vi "Loop_Overlord.vi"() -> ()   [LabVIEW 2017, in "Rotation_Overlord.lvlib"]
uses:
  Rotation_Overlord.lvlib
  CLUSTER_Rotation_CMD.ctl
  ENUM_Rotation_Positon.ctl
  TypeDef/CLUSTER_Overlord_Systems.ctl
  Arm/CLUSTER_CMD_SM_Lift_Rotate.ctl
  Arm/ENUM_SM_Rotate_Positions.ctl
  Claw Rotation/CLUSTER_CMD_SM_Lift_Rotate.ctl
  Claw Rotation/ENUM_SM_Rotate_Positions.ctl
  Lift/CLUSTER_CMD_SM_Lift_Rotate.ctl
  Lift/ENUM_SM_Rotate_Positions.ctl
  ENUM_Overloard_State.ctl
  Arm/ENUM_SM_State.ctl
  Claw Rotation/ENUM_SM_State.ctl
  Lift/ENUM_SM_State.ctl
  Lift/CLUSTER_ACT_Lift Output.ctl
  _SHARE ALL/RoboRio Share All/SRX Share All/TypeDefs SRX/Cluster_SRX_General Data.ctl
  _SHARE ALL/RoboRio Share All/SRX Share All/TypeDefs SRX/Cluster_SRX_Common Runtime Data.ctl
  _SHARE ALL/RoboRio Share All/SRX Share All/TypeDefs SRX/Cluster_SRX_Error Calculations.ctl
  _SHARE ALL/RoboRio Share All/SRX Share All/TypeDefs SRX/Cluster_SRX_Voltage Out Data.ctl
  _SHARE ALL/RoboRio Share All/SRX Share All/TypeDefs SRX/Cluster_SRX_Sensor Out Data.ctl
  _SHARE ALL/RoboRio Share All/SRX Share All/TypeDefs SRX/Cluster_SRX_Sensor Quad Data.ctl
  _SHARE ALL/RoboRio Share All/SRX Share All/TypeDefs SRX/Cluster_SRX_Analog In Data.ctl
  _SHARE ALL/RoboRio Share All/SRX Share All/TypeDefs SRX/Cluster_SRX_PWM Sensor Data.ctl
  _SHARE ALL/RoboRio Share All/SRX Share All/TypeDefs SRX/Cluster_SRX_F and R Limit Indicators.ctl
  ENUM_Overloard_Action.ctl
  _SHARE ALL/Global Share All/Global_STOP.vi
  Global_CMD.vi
  Arm/Global_SM Write_Data Out.vi
  Claw Rotation/Global_SM Write_Data Out.vi
  Lift/Global_SM Write_Data Out.vi
  Lift/Global_ACT Write_Data Out.vi
  Lift/Global_CMD.vi
  Claw Rotation/Global_CMD.vi
  Arm/Global_CMD.vi
  Arm/Arm.lvlib
  Claw Rotation/Claw_Rotation.lvlib
  Lift/Lift.lvlib
panel:
  out "State":T1
  out "Stage Counter":i32
  out "Lift CMD":T2={"Enable System"=TRUE, "Rotate Position"=enum."Neutral: 0", "Manual Velocity"=0.0, "Manual Mode"=FALSE, "Manual Override"=FALSE}
  out "Claw Rotation CMD":T4={"Enable System"=TRUE, "Rotate Position"=enum."Neutral: -500", "Manual Velocity"=0.0, "Manual Mode"=FALSE, "Manual Override"=FALSE}
  out "Arm CMD":T6={"Enable System"=TRUE, "Rotate Position"=enum."Neutral: 3230", "Manual Velocity"=0.0, "Manual Mode"=FALSE, "Manual Override"=FALSE}
  out "Rotation CMD":T8={"Rotation Positon"=enum."Neutral", "Enable Rotation"=TRUE, "Manual Override"=FALSE, "Arm Value"=0.0, "Claw Rotation Value"=0.0, "Lift Value"=0.0, "Enable"={"Lift"=FALSE, "Arm"=FALSE, "Claw Rotation"=FALSE}}
  out "Cycle Time (S)":dbl format="%.3g"
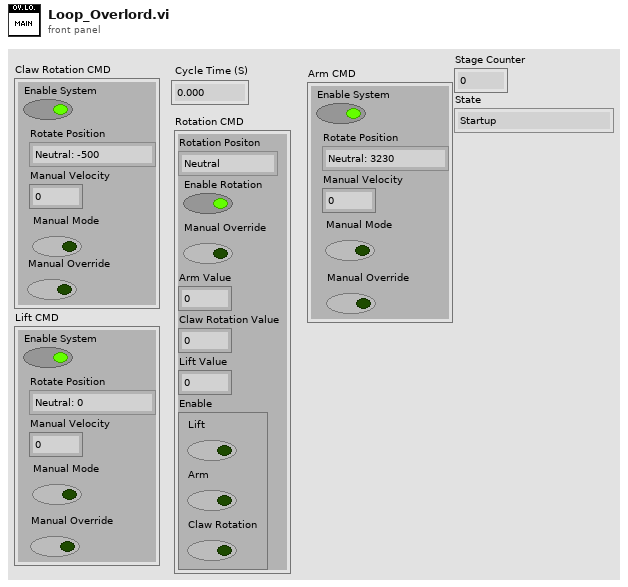
[diagram p1: front panel]
types:
  T1 = typedef "Rotation_Overlord.lvlib/ENUM_Overloard_State.ctl" = enum16{"Startup", "Idle", "Neutral - Moving", "Neutral - Holding", "Pickup - Moving", "Pickup - Holding", "Switch - Moving", "Switch - Holding", "Scale - Moving", "Scale - Holding", "Climb - Moving", "Climb - Holding", "F_Manual", "Manual", "Shutdown"}
  T2 = typedef "Lift.lvlib/CLUSTER_CMD_SM_Lift_Rotate.ctl" = cluster{"Enable System":bool, "Rotate Position":T3, "Manual Velocity":dbl, "Manual Mode":bool, "Manual Override":bool}
  T3 = typedef "Lift.lvlib/ENUM_SM_Rotate_Positions.ctl" = enum16{"Neutral: 0", "Pickup: 0", "Switch: 0", "Scale:  117000", "Climb: 0"}
  T4 = typedef "Claw_Rotation.lvlib/CLUSTER_CMD_SM_Lift_Rotate.ctl" = cluster{"Enable System":bool, "Rotate Position":T5, "Manual Velocity":dbl, "Manual Mode":bool, "Manual Override":bool}
  T5 = typedef "Claw_Rotation.lvlib/ENUM_SM_Rotate_Positions.ctl" = enum16{"Neutral: -500", "Pickup: -700", "Switch: -700", "Scale: 0", "Climb: 0"}
  T6 = typedef "Arm.lvlib/CLUSTER_CMD_SM_Lift_Rotate.ctl" = cluster{"Enable System":bool, "Rotate Position":T7, "Manual Velocity":dbl, "Manual Mode":bool, "Manual Override":bool}
  T7 = typedef "Arm.lvlib/ENUM_SM_Rotate_Positions.ctl" = enum16{"Neutral: 3230", "Pickup: 0", "Switch: 2100", "Scale: 3700", "Climb: 0"}
  T8 = typedef "Rotation_Overlord.lvlib/CLUSTER_Rotation_CMD.ctl" = cluster{"Rotation Positon":T9, "Enable Rotation":bool, "Manual Override":bool, "Arm Value":dbl, "Claw Rotation Value":dbl, "Lift Value":dbl, "Enable":T10}
  T9 = typedef "Rotation_Overlord.lvlib/ENUM_Rotation_Positon.ctl" = enum16{"Neutral", "Pickup", "Switch", "Scale", "Climb", "Manual"}
  T10 = typedef "CLUSTER_Overlord_Systems.ctl" = cluster{"Lift":bool, "Arm":bool, "Claw Rotation":bool}
  T11 = typedef "Lift.lvlib/CLUSTER_ACT_Lift Output.ctl" = cluster{"Device Info Out":T12, "Common Runtime Data Out":T13, "Quad Sensor Data Out":T17, "Analog Sensor Data Out":T18, "PWM Data Out":T19, "Hard Limits Out":T20}
  T12 = typedef "Cluster_SRX_General Data.ctl" = cluster{"Device ID":i32, "Firmware Version":i32, "Inverted?":bool, "Has Reset Occurred?":bool}
  T13 = typedef "Cluster_SRX_Common Runtime Data.ctl" = cluster{"Calc":T14, "Voltage ":T15, "Sensor":T16, "Current":dbl, "Temp":dbl}
  T14 = typedef "Cluster_SRX_Error Calculations.ctl" = cluster{"Error":i32, "D-Error":dbl, "I-Acc":dbl}
  T15 = typedef "Cluster_SRX_Voltage Out Data.ctl" = cluster{"Percent":dbl, "Output":dbl, "Bus":dbl}
  T16 = typedef "Cluster_SRX_Sensor Out Data.ctl" = cluster{"Pos":i32, "Vel":i32}
  T17 = typedef "Cluster_SRX_Sensor Quad Data.ctl" = cluster{"Position":i32, "Velocity":i32, "Quad A Pin":bool, "Quad B Pin":bool, "Quad Idx Pin":bool}
  T18 = typedef "Cluster_SRX_Analog In Data.ctl" = cluster{"WithOv":i32, "Raw":i32, "Velocity":i32}
  T19 = typedef "Cluster_SRX_PWM Sensor Data.ctl" = cluster{"Position":i32, "Velocity":i32, "High(us)":i32, "Period(us)":i32}
  T20 = typedef "Cluster_SRX_F and R Limit Indicators.ctl" = cluster{"Forward Closed?":bool, "Reverse Closed?":bool}
  T21 = typedef "Lift.lvlib/ENUM_SM_State.ctl" = enum16{"Startup", "Idle", "F_Manual", "Manual", "Position - Moving", "Position - Holding", "Shutdown"}
  T22 = typedef "Claw_Rotation.lvlib/ENUM_SM_State.ctl" = enum16{"Startup", "Idle", "F_Manual", "Manual", "Position - Moving", "Position - Holding", "Shutdown"}
  T23 = typedef "Arm.lvlib/ENUM_SM_State.ctl" = enum16{"Startup", "Idle", "F_Manual", "Manual", "Position - Moving", "Position - Holding", "Shutdown"}
  T24 = typedef "Rotation_Overlord.lvlib/ENUM_Overloard_Action.ctl" = enum16{"No Action", "Reset Time", "Disable All", "Disable Lift", "Disable Arm", "Disable Claw Rotation", "Enable Lift", "Enable Arm", "Enable Claw Rotation", "Enable All", "Set Starting/Neutral", "Set Pickup/Exchange", "Set Switch", "Set Scale", "Set Climb", "Manual All", "Manual Arm", "Manual Lift", "Manual Claw Rotation", "Manual Off Arm", "Manual Off Lift", "Manual Off Claw Rotation", "Manual Off All", "Reset Stage Counter", "Increment Counter", "Manual Override", "Manual Override Off", "Netural Path - Arm First", "Neutral Path - Normal"}
  T25 = cluster{"State":T1, "Previous State":T1, "Current Time":timestamp, "Previous Time":timestamp, "Start Time":timestamp, "Target Time (ms)":u32, "Cycle Time(S)":dbl, "Arm CMD":T6, "Claw Rotation CMD":T4, "Lift CMD":T2, "Rotation CMD":T8, "Arm State":T23, "Claw Rotation State":T22, "Lift State":T21, "Stage Counter":i32, "Previous Rotation CMD":T8, "Neutral Path":bool, "Lift Data":T11}
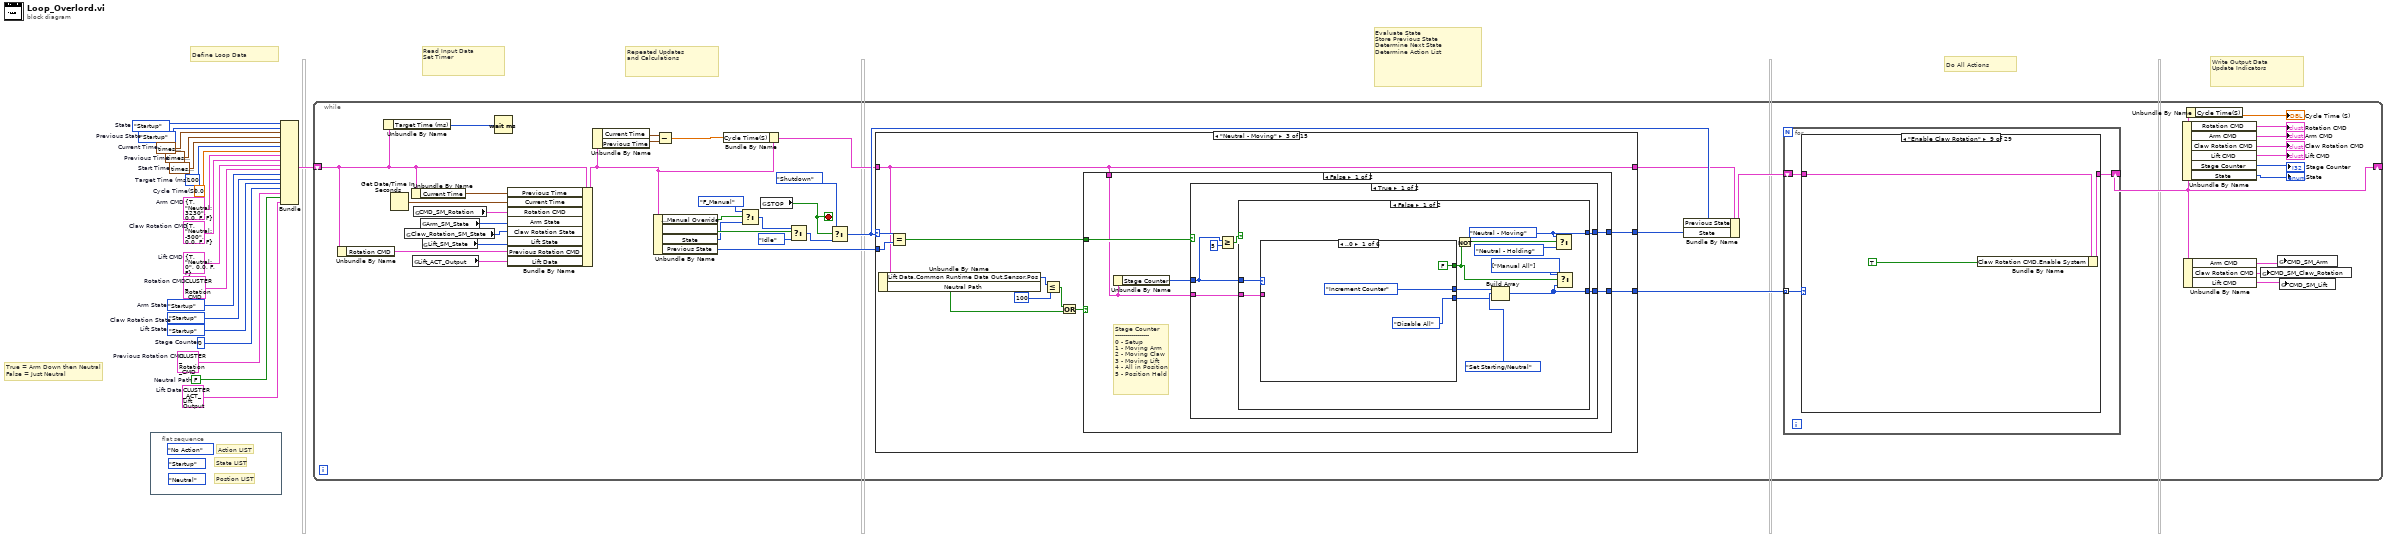
[diagram p0: block diagram]
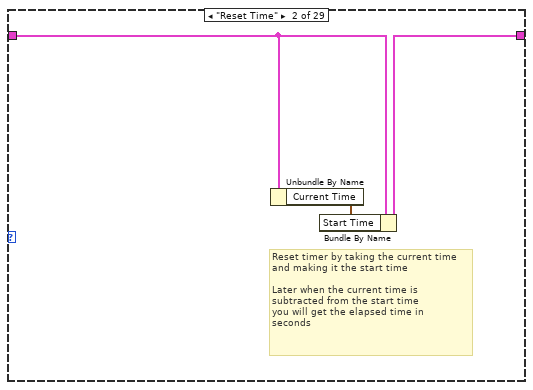
[diagram p3: hidden frame]
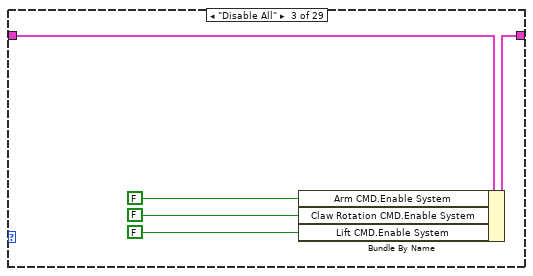
[diagram p4: hidden frame]
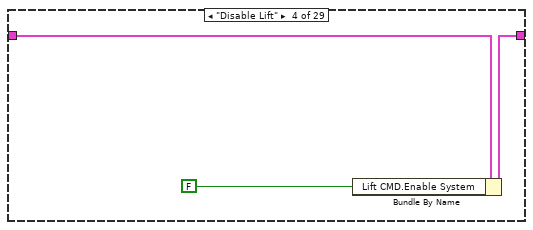
[diagram p5: hidden frame]
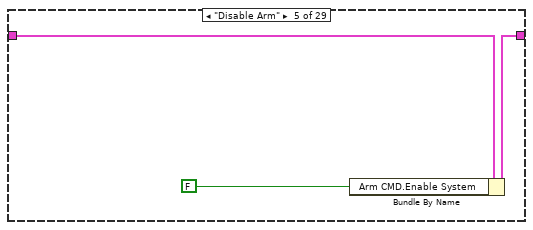
[diagram p6: hidden frame]
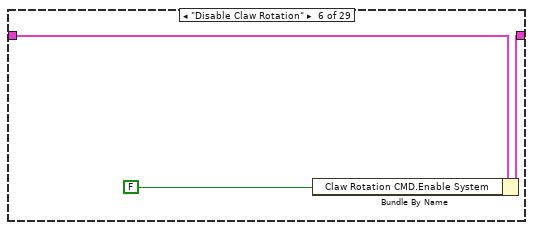
[diagram p7: hidden frame]
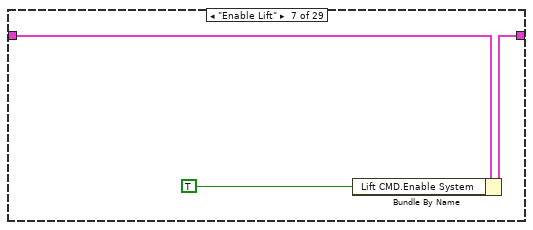
[diagram p8: hidden frame]
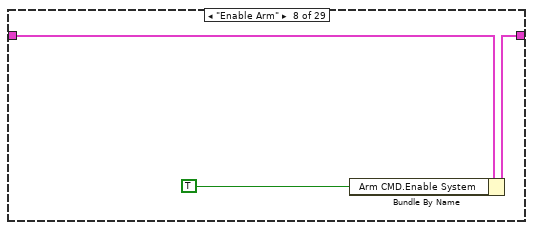
[diagram p9: hidden frame]
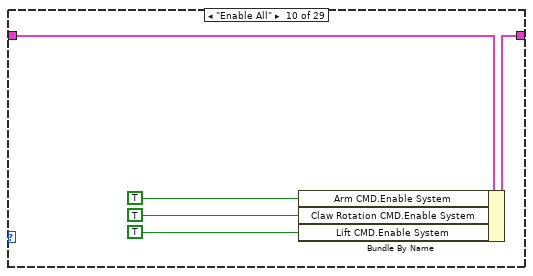
[diagram p10: hidden frame]
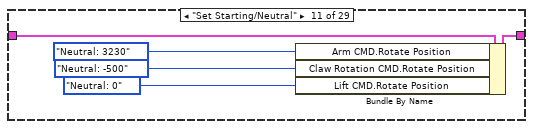
[diagram p11: hidden frame]
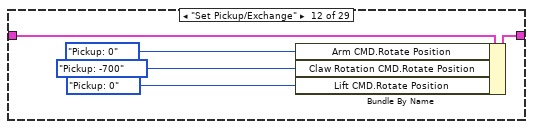
[diagram p12: hidden frame]
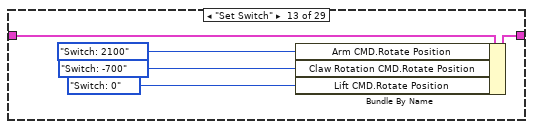
[diagram p13: hidden frame]
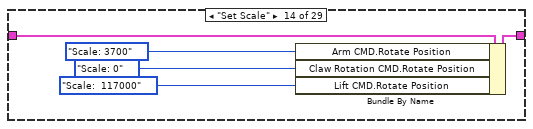
[diagram p14: hidden frame]
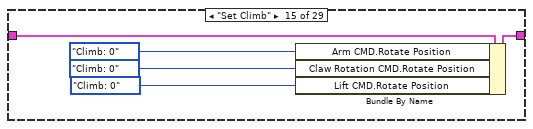
[diagram p15: hidden frame]
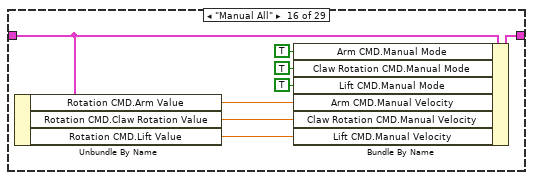
[diagram p16: hidden frame]
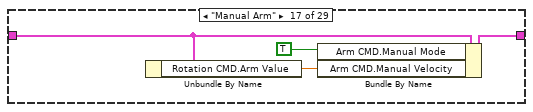
[diagram p17: hidden frame]
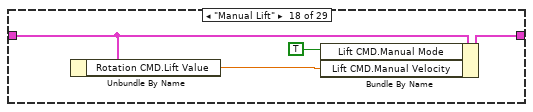
[diagram p18: hidden frame]
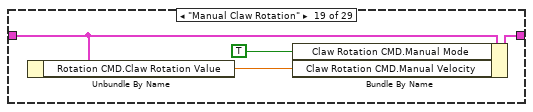
[diagram p19: hidden frame]
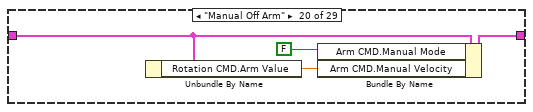
[diagram p20: hidden frame]
diagram:
  w1 = T11 {"Device Info Out"={"Device ID"=0, "Firmware Version"=0, "Inverted?"=FALSE, "Has Reset Occurred?"=FALSE}, "Common Runtime Data Out"={"Calc"={"Error"=0, "D-Error"=0.0, "I-Acc"=0.0}, "Voltage "={"Percent"=0.0, "Output"=0.0, "Bus"=0.0}, "Sensor"={"Pos"=0, "Vel"=0}, "Current"=0.0, "Temp"=0.0}, "Quad Sensor Data Out"={"Position"=0, "Velocity"=0, "Quad A Pin"=FALSE, "Quad B Pin"=FALSE, "Quad Idx Pin"=FALSE}, "Analog Sensor Data Out"={"WithOv"=0, "Raw"=0, "Velocity"=0}, "PWM Data Out"={"Position"=0, "Velocity"=0, "High(us)"=0, "Period(us)"=0}, "Hard Limits Out"={"Forward Closed?"=FALSE, "Reverse Closed?"=FALSE}}  # Lift Data
  w2 = FALSE  # Neutral Path
  w3 = T8 {"Rotation Positon"=enum."Neutral", "Enable Rotation"=TRUE, "Manual Override"=FALSE, "Arm Value"=0.0, "Claw Rotation Value"=0.0, "Lift Value"=0.0, "Enable"={"Lift"=FALSE, "Arm"=FALSE, "Claw Rotation"=FALSE}}  # Previous Rotation CMD
  w4 = 0  # Stage Counter
  w5 = ENUM_SM_State."Startup"  # Lift State
  w6 = ENUM_SM_State."Startup"  # Claw Rotation State
  w7 = ENUM_SM_State."Startup"  # Arm State
  w8 = T8 {"Rotation Positon"=enum."Neutral", "Enable Rotation"=TRUE, "Manual Override"=FALSE, "Arm Value"=0.0, "Claw Rotation Value"=0.0, "Lift Value"=0.0, "Enable"={"Lift"=FALSE, "Arm"=FALSE, "Claw Rotation"=FALSE}}  # Rotation CMD
  w9 = T2 {"Enable System"=TRUE, "Rotate Position"=enum."Neutral: 0", "Manual Velocity"=0.0, "Manual Mode"=FALSE, "Manual Override"=FALSE}  # Lift CMD
  w10 = T4 {"Enable System"=TRUE, "Rotate Position"=enum."Neutral: -500", "Manual Velocity"=0.0, "Manual Mode"=FALSE, "Manual Override"=FALSE}  # Claw Rotation CMD
  w11 = T6 {"Enable System"=TRUE, "Rotate Position"=enum."Neutral: 3230", "Manual Velocity"=0.0, "Manual Mode"=FALSE, "Manual Override"=FALSE}  # Arm CMD
  w12 = 0.0  # Cycle Time(S)
  w13 = ENUM_Overloard_State."Startup"  # Previous State
  w14 = timestamp(0 s since 1904-01-01)  # Previous Time
  w15 = u32 100  # Target Time (ms)
  w16 = timestamp(0 s since 1904-01-01)  # Start Time
  w17 = timestamp(0 s since 1904-01-01)  # Current Time
  w18 = ENUM_Overloard_State."Startup"  # State
  # "True = Arm Down then Neutral\nFalse = Just Neutral"
  # "Define Loop Data"
  # "Repeated Updates\nand Calculations"
  # "Read Input Data\nSet Timer"
  # "Evaluate State\nStore Previous State\nDetermine Next State\nDetermine Action List"
  # "Do All Actions"
  # "Write Output Data\nUpdate Indicators"
  n1 = flat-sequence {
    frame #0 {
      (unwired) ENUM_Rotation_Positon."Neutral" ("Rotation Position")
      (unwired) ENUM_Overloard_State."Startup" ("State")
      (unwired) ENUM_Overloard_Action."No Action" ("Action")
      # "Postion LIST"
      # "State LIST"
      # "Action LIST"
    }
  }
  n2 = Bundle("State"=w18, "Previous State"=w13, "Current Time"=w17, "Previous Time"=w14, "Start Time"=w16, "Target Time (ms)"=w15, "Cycle Time(S)"=w12, "Arm CMD"=w11, "Claw Rotation CMD"=w10, "Lift CMD"=w9, "Rotation CMD"=w8, "Arm State"=w7, "Claw Rotation State"=w6, "Lift State"=w5, "Stage Counter"=w4, "Previous Rotation CMD"=w3, "Neutral Path"=w2, "Lift Data"=w1) -> (w19:T25)  [unwired: 1 in]
  n3 = while {
    shift-right: [w53] -> _
    shift-left: w19 -> [w22]
    stop <- w43 stop-if-true
    n4 = Unbundle By Name(w22) -> ("Rotation CMD"=w21:T8)
    n5 = Unbundle By Name(w22) -> ("Target Time (ms)"=w57:u32)
    n6 = Get Date/Time In Seconds() -> (seconds since 1Jan1904=w60:timestamp)
    n7 = global read "Global_SM Write_Data Out.vi" "Claw_Rotation_SM_State"() -> (w40:T22)
    n8 = Unbundle By Name(w22) -> ("Current Time"=w56:timestamp)
    n9 = global read "Global_ACT Write_Data Out.vi" "Lift_ACT_Output"() -> (w20:T11)
    n10 = global read "Global_CMD.vi" "CMD_SM_Rotation"() -> (w42:T8)
    n11 = global read "Global_SM Write_Data Out.vi" "Arm_SM_State"() -> (w41:T23)
    n12 = global read "Global_SM Write_Data Out.vi" "Lift_SM_State"() -> (w39:T21)
    n13 = Wait (ms)(milliseconds to wait=w57) -> ()  [unwired: 1 out]
    n14 = Bundle By Name(cluster=w22, "Previous Time"=w56, "Current Time"=w60, "Rotation CMD"=w42, "Arm State"=w41, "Claw Rotation State"=w40, "Lift State"=w39, "Previous Rotation CMD"=w21, "Lift Data"=w20) -> (w49:T25)
    n15 = Unbundle By Name(w49) -> ("Current Time"=w50:timestamp, "Previous Time"=w51:timestamp)
    n16 = Unbundle By Name(w49) -> ("Rotation CMD.Manual Override"=w33:bool, "Rotation CMD.Enable Rotation"=w35:bool, "State"=w34:T1, "Previous State"=w55:T1)
    n17 = Subtract(x=w50, y=w51) -> (x-y=w47:dbl)
    n18 = Bundle By Name(cluster=w49, "Cycle Time(S)"=w47) -> (w48:T25)
    n19 = Select(t=ENUM_Overloard_State."F_Manual", s=w33, f=w34) -> (s? t:f=w26:T1)
    n20 = global read "Global_STOP.vi" "STOP"() -> (w43:bool)
    n21 = Select(t=w26, s=w35, f=ENUM_Overloard_State."Idle" ("t")) -> (s? t:f=w36:T1)
    n22 = Select(t=ENUM_Overloard_State."Shutdown" ("State"), s=w43, f=w36) -> (s? t:f=w54:T1)
    n23 = case shown="\"Neutral - Moving\"" w54 {
      selector: w54 -> [_ _ w223 _ w401 _ w474 _ w547 _ w655 _ _ _ _]
      tunnel: w48 -> [w182 w188 w218 w394 w395 w467 w468 w540 w541 w648 w649 w720 w723 w729 w736]
      tunnel: [w182 w188 w218 w394 w395 w467 w468 w540 w541 w648 w649 w720 w723 w729 w736] -> w27
      tunnel: w55 -> [_ w185 w222 _ w400 _ w473 _ w546 _ w654 _ _ _ _]
      tunnel: [w180 w187 w219 w392 w397 w465 w470 w538 w543 w646 w651 w718 w721 w725 w735] -> w38
      tunnel: [ENUM_Overloard_State."Idle" ("State") w186 w220 ENUM_Overloard_State."Manual" ("State") w398 ENUM_Overloard_State."Manual" ("State") w471 ENUM_Overloard_State."Manual" ("State") w544 ENUM_Overloard_State."Manual" ("State") w652 ENUM_Overloard_State."Manual" ("State") ENUM_Overloard_State."Manual" ("State") w724 ENUM_Overloard_State."Shutdown" ("State")] -> w37
      frame "Startup" {
        w180 = T24[] [enum."Disable All", enum."Reset Time", enum."Reset Stage Counter"] items=["No Action", "Reset Time", "Disable All", "Disable Lift", "Disable Arm", "Disable Claw Rotation", "Enable Lift", "Enable Arm", "Enable Claw Rotation", "Enable All", "Set Starting/Neutral", "Set Pickup/Exchange", "Set Switch", "Set Scale", "Set Climb", "Manual All", "Manual Arm", "Manual Lift", "Manual Claw Rotation", "Manual Off Arm", "Manual Off Lift", "Manual Off Claw Rotation", "Manual Off All", "Reset Stage Counter", "Increment Counter", "Manual Override", "Manual Override Off", "Netural Path - Arm First", "Neutral Path - Normal"] ("Actions")
      }
      frame "Idle" {
        n24 = Equal?(x=w185, y=ENUM_Overloard_State."F_Manual") -> (x = y?=w183:bool)
        n25 = case shown="False" w183 {
          tunnel: w188 -> [_ w195]
          tunnel: [w189 w194] -> w187
          tunnel: [ENUM_Overloard_State."Idle" ("State") w192] -> w186
          frame True {
            w189 = T24[] [enum."Manual Override Off"] items=["No Action", "Reset Time", "Disable All", "Disable Lift", "Disable Arm", "Disable Claw Rotation", "Enable Lift", "Enable Arm", "Enable Claw Rotation", "Enable All", "Set Starting/Neutral", "Set Pickup/Exchange", "Set Switch", "Set Scale", "Set Climb", "Manual All", "Manual Arm", "Manual Lift", "Manual Claw Rotation", "Manual Off Arm", "Manual Off Lift", "Manual Off Claw Rotation", "Manual Off All", "Reset Stage Counter", "Increment Counter", "Manual Override", "Manual Override Off", "Netural Path - Arm First", "Neutral Path - Normal"] ("Actions")
          }
          frame False {
            n26 = Unbundle By Name(w195) -> ("Rotation CMD.Rotation Positon"=w193:T9, "Rotation CMD.Enable Rotation"=w191:bool)
            n27 = case shown="True" w191 {
              tunnel: [w197 w212] -> w194
              tunnel: w193 -> [w198 _]
              tunnel: [w196 ENUM_Overloard_State."Idle" ("State")] -> w192
              frame True {
                n28 = case shown="\"Pickup\"" w198 {
                  tunnel: [w200 w202 w204 w206 w208 w210] -> w197
                  tunnel: [ENUM_Overloard_State."Neutral - Moving" ("State") ENUM_Overloard_State."Pickup - Moving" ("State") ENUM_Overloard_State."Switch - Moving" ("State") ENUM_Overloard_State."Scale - Moving" ("State") ENUM_Overloard_State."Climb - Moving" ("State") ENUM_Overloard_State."Manual" ("State")] -> w196
                  frame "Neutral" {
                    w200 = T24[] [enum."Set Starting/Neutral"] items=["No Action", "Reset Time", "Disable All", "Disable Lift", "Disable Arm", "Disable Claw Rotation", "Enable Lift", "Enable Arm", "Enable Claw Rotation", "Enable All", "Set Starting/Neutral", "Set Pickup/Exchange", "Set Switch", "Set Scale", "Set Climb", "Manual All", "Manual Arm", "Manual Lift", "Manual Claw Rotation", "Manual Off Arm", "Manual Off Lift", "Manual Off Claw Rotation", "Manual Off All", "Reset Stage Counter", "Increment Counter", "Manual Override", "Manual Override Off", "Netural Path - Arm First", "Neutral Path - Normal"] ("Actions")
                  }
                  frame "Pickup" {
                    w202 = T24[] [enum."Set Pickup/Exchange"] items=["No Action", "Reset Time", "Disable All", "Disable Lift", "Disable Arm", "Disable Claw Rotation", "Enable Lift", "Enable Arm", "Enable Claw Rotation", "Enable All", "Set Starting/Neutral", "Set Pickup/Exchange", "Set Switch", "Set Scale", "Set Climb", "Manual All", "Manual Arm", "Manual Lift", "Manual Claw Rotation", "Manual Off Arm", "Manual Off Lift", "Manual Off Claw Rotation", "Manual Off All", "Reset Stage Counter", "Increment Counter", "Manual Override", "Manual Override Off", "Netural Path - Arm First", "Neutral Path - Normal"] ("Actions")
                  }
                  frame "Switch" {
                    w204 = T24[] [enum."Set Switch"] items=["No Action", "Reset Time", "Disable All", "Disable Lift", "Disable Arm", "Disable Claw Rotation", "Enable Lift", "Enable Arm", "Enable Claw Rotation", "Enable All", "Set Starting/Neutral", "Set Pickup/Exchange", "Set Switch", "Set Scale", "Set Climb", "Manual All", "Manual Arm", "Manual Lift", "Manual Claw Rotation", "Manual Off Arm", "Manual Off Lift", "Manual Off Claw Rotation", "Manual Off All", "Reset Stage Counter", "Increment Counter", "Manual Override", "Manual Override Off", "Netural Path - Arm First", "Neutral Path - Normal"] ("Actions")
                  }
                  frame "Scale" {
                    w206 = T24[] [enum."Set Scale"] items=["No Action", "Reset Time", "Disable All", "Disable Lift", "Disable Arm", "Disable Claw Rotation", "Enable Lift", "Enable Arm", "Enable Claw Rotation", "Enable All", "Set Starting/Neutral", "Set Pickup/Exchange", "Set Switch", "Set Scale", "Set Climb", "Manual All", "Manual Arm", "Manual Lift", "Manual Claw Rotation", "Manual Off Arm", "Manual Off Lift", "Manual Off Claw Rotation", "Manual Off All", "Reset Stage Counter", "Increment Counter", "Manual Override", "Manual Override Off", "Netural Path - Arm First", "Neutral Path - Normal"] ("Actions")
                  }
                  frame "Climb" {
                    w208 = T24[] [enum."Set Climb"] items=["No Action", "Reset Time", "Disable All", "Disable Lift", "Disable Arm", "Disable Claw Rotation", "Enable Lift", "Enable Arm", "Enable Claw Rotation", "Enable All", "Set Starting/Neutral", "Set Pickup/Exchange", "Set Switch", "Set Scale", "Set Climb", "Manual All", "Manual Arm", "Manual Lift", "Manual Claw Rotation", "Manual Off Arm", "Manual Off Lift", "Manual Off Claw Rotation", "Manual Off All", "Reset Stage Counter", "Increment Counter", "Manual Override", "Manual Override Off", "Netural Path - Arm First", "Neutral Path - Normal"] ("Actions")
                  }
                  frame "Manual" {
                    w210 = T24[] [enum."No Action"] items=["No Action", "Reset Time", "Disable All", "Disable Lift", "Disable Arm", "Disable Claw Rotation", "Enable Lift", "Enable Arm", "Enable Claw Rotation", "Enable All", "Set Starting/Neutral", "Set Pickup/Exchange", "Set Switch", "Set Scale", "Set Climb", "Manual All", "Manual Arm", "Manual Lift", "Manual Claw Rotation", "Manual Off Arm", "Manual Off Lift", "Manual Off Claw Rotation", "Manual Off All", "Reset Stage Counter", "Increment Counter", "Manual Override", "Manual Override Off", "Netural Path - Arm First", "Neutral Path - Normal"] ("Actions")
                  }
                }
              }
              frame False {
                w212 = T24[] [enum."Disable All"] items=["No Action", "Reset Time", "Disable All", "Disable Lift", "Disable Arm", "Disable Claw Rotation", "Enable Lift", "Enable Arm", "Enable Claw Rotation", "Enable All", "Set Starting/Neutral", "Set Pickup/Exchange", "Set Switch", "Set Scale", "Set Climb", "Manual All", "Manual Arm", "Manual Lift", "Manual Claw Rotation", "Manual Off Arm", "Manual Off Lift", "Manual Off Claw Rotation", "Manual Off All", "Reset Stage Counter", "Increment Counter", "Manual Override", "Manual Override Off", "Netural Path - Arm First", "Neutral Path - Normal"] ("Actions")
              }
            }
          }
        }
      }
      frame "Neutral - Moving" {
        n29 = Unbundle By Name(w218) -> ("Lift Data.Common Runtime Data Out.Sensor.Pos"=w214:i32, "Neutral Path"=w216:bool)
        n30 = Equal?(x=w223, y=w222) -> (x = y?=w221:bool)
        n31 = Less Or Equal?(x=w214, y=100) -> (x <= y?=w215:bool)
        n32 = Or(x=w215, y=w216) -> (x .or. y?=w217:bool)
        n33 = case shown="False" w217 {
          tunnel: w221 -> [w228 w301]
          tunnel: [w227 w300] -> w220
          tunnel: [w226 w299] -> w219
          tunnel: w218 -> [w224 w297]
          frame False {
            # "Stage Counter\n-----------------\n0 - Setup\n1 - Moving Arm\n2 - Moving Claw\n3 - Moving Lift\n4 - All in Position\n5 - Position Held"
            n34 = Unbundle By Name(w224) -> ("Stage Counter"=w225:i32)
            n35 = case shown="True" w228 {
              tunnel: [w232 ENUM_Overloard_State."Neutral - Moving" ("State")] -> w227
              tunnel: [w231 w295] -> w226
              tunnel: w225 -> [w230 _]
              tunnel: w224 -> [w229 _]
              frame True {
                n36 = Greater Or Equal?(x=w230, y=5) -> (x >= y?=w233:bool)
                n37 = case shown="False" w233 {
                  tunnel: [w241 ENUM_Overloard_State."Neutral - Holding" ("State")] -> w232
                  tunnel: [w240 w293] -> w231
                  tunnel: w230 -> [w245 _]
                  tunnel: w229 -> [w242 _]
                  frame False {
                    w239 = T24[] [enum."Manual All"] items=["No Action", "Reset Time", "Disable All", "Disable Lift", "Disable Arm", "Disable Claw Rotation", "Enable Lift", "Enable Arm", "Enable Claw Rotation", "Enable All", "Set Starting/Neutral", "Set Pickup/Exchange", "Set Switch", "Set Scale", "Set Climb", "Manual All", "Manual Arm", "Manual Lift", "Manual Claw Rotation", "Manual Off Arm", "Manual Off Lift", "Manual Off Claw Rotation", "Manual Off All", "Reset Stage Counter", "Increment Counter", "Manual Override", "Manual Override Off", "Netural Path - Arm First", "Neutral Path - Normal"] ("t")
                    w241 = ENUM_Overloard_State."Neutral - Moving" ("State")
                    n38 = case shown="..0" w245 {
                      tunnel: [ENUM_Overloard_Action."Increment Counter" ("Action") w253 w262 w271 w289 w291] -> w244
                      tunnel: w242 -> [_ w257 w266 w275 w290 _]
                      tunnel: [FALSE FALSE FALSE FALSE FALSE TRUE] -> w237
                      tunnel: [ENUM_Overloard_Action."Disable All" ("Action") ENUM_Overloard_Action."No Action" ("Action") ENUM_Overloard_Action."No Action" ("Action") ENUM_Overloard_Action."No Action" ("Action") ENUM_Overloard_Action."No Action" ("Action") w291] -> w235
                      frame ..0 {
                      }
                      frame 1 {
                        n39 = Unbundle By Name(w257) -> ("Arm State"=w256:T23)
                        n40 = Equal?(x=w256, y=ENUM_SM_State."Position - Holding") -> (x = y?=w254:bool)
                        n41 = Select(t=ENUM_Overloard_Action."Increment Counter", s=w254, f=ENUM_Overloard_Action."Enable Arm" ("Action")) -> (s? t:f=w253:T24)
                      }
                      frame 2 {
                        n42 = Unbundle By Name(w266) -> ("Claw Rotation State"=w265:T22)
                        n43 = Equal?(x=w265, y=ENUM_SM_State."Position - Holding") -> (x = y?=w263:bool)
                        n44 = Select(t=ENUM_Overloard_Action."Increment Counter", s=w263, f=ENUM_Overloard_Action."Enable Claw Rotation" ("Action")) -> (s? t:f=w262:T24)
                      }
                      frame 3 {
                        n45 = Unbundle By Name(w275) -> ("Lift State"=w274:T21)
                        n46 = Equal?(x=w274, y=ENUM_SM_State."Position - Holding") -> (x = y?=w272:bool)
                        n47 = Select(t=ENUM_Overloard_Action."Increment Counter", s=w272, f=ENUM_Overloard_Action."Enable Lift" ("Action")) -> (s? t:f=w271:T24)
                      }
                      frame 4 {
                        w286 = ENUM_SM_State."Position - Holding" ("y")
                        n48 = Unbundle By Name(w290) -> ("Lift State"=w285:T21, "Arm State"=w284:T23, "Claw Rotation State"=w283:T22)
                        n49 = Equal?(x=w286, y=w285) -> (x = y?=w282:bool)
                        n50 = Equal?(x=w286, y=w284) -> (x = y?=w281:bool)
                        n51 = Equal?(x=w286, y=w283) -> (x = y?=w279:bool)
                        n52 = And(x=w282, y=w281) -> (x .and. y?=w280:bool)
                        n53 = And(x=w280, y=w279) -> (x .and. y?=w278:bool)
                        n54 = Select(t=ENUM_Overloard_Action."Increment Counter", s=w278, f=ENUM_Overloard_Action."Enable All" ("Action")) -> (s? t:f=w289:T24)
                      }
                      frame 5.. {
                        w291 = ENUM_Overloard_Action."No Action" ("Action")
                      }
                    }
                    n55 = Not(x=w237) -> (.not. x?=w236:bool)
                    n56 = Build Array(w244, ENUM_Overloard_Action."Set Starting/Neutral" ("Action"), w235) -> (w240:T24[])
                    n57 = Select(t=w241, s=w236, f=ENUM_Overloard_State."Neutral - Holding") -> ()  [unwired: 1 out]
                    n58 = Select(t=w239, s=w237, f=w240) -> ()  [unwired: 1 out]
                  }
                  frame True {
                    w293 = T24[] [] items=["No Action", "Reset Time", "Disable All", "Disable Lift", "Disable Arm", "Disable Claw Rotation", "Enable Lift", "Enable Arm", "Enable Claw Rotation", "Enable All", "Set Starting/Neutral", "Set Pickup/Exchange", "Set Switch", "Set Scale", "Set Climb", "Manual All", "Manual Arm", "Manual Lift", "Manual Claw Rotation", "Manual Off Arm", "Manual Off Lift", "Manual Off Claw Rotation", "Manual Off All", "Reset Stage Counter", "Increment Counter", "Manual Override", "Manual Override Off", "Netural Path - Arm First", "Neutral Path - Normal"] ("Actions")
                  }
                }
              }
              frame False {
                w295 = T24[] [enum."Set Starting/Neutral", enum."Manual All", enum."Reset Stage Counter", enum."Neutral Path - Normal"] items=["No Action", "Reset Time", "Disable All", "Disable Lift", "Disable Arm", "Disable Claw Rotation", "Enable Lift", "Enable Arm", "Enable Claw Rotation", "Enable All", "Set Starting/Neutral", "Set Pickup/Exchange", "Set Switch", "Set Scale", "Set Climb", "Manual All", "Manual Arm", "Manual Lift", "Manual Claw Rotation", "Manual Off Arm", "Manual Off Lift", "Manual Off Claw Rotation", "Manual Off All", "Reset Stage Counter", "Increment Counter", "Manual Override", "Manual Override Off", "Netural Path - Arm First", "Neutral Path - Normal"] ("Actions")
              }
            }
          }
          frame True {
            # "Stage Counter\n-----------------\n0 - Setup\n1 - Move Claw  - Down\n2 - Move Arm - Down\n3 - Setup Neutral\n4 - Moving Arm\n5 - Moving Claw\n6 - Moving Lift\n7 - All in Position\n8 - Position Held"
            n59 = Unbundle By Name(w297) -> ("Stage Counter"=w298:i32)
            n60 = case shown="True" w301 {
              tunnel: [w305 ENUM_Overloard_State."Neutral - Moving" ("State")] -> w300
              tunnel: [w304 w390] -> w299
              tunnel: w298 -> [w303 _]
              tunnel: w297 -> [w302 _]
              frame True {
                n61 = Greater Or Equal?(x=w303, y=8) -> (x >= y?=w306:bool)
                n62 = case shown="False" w306 {
                  tunnel: [w315 ENUM_Overloard_State."Neutral - Holding" ("State")] -> w305
                  tunnel: [w314 w388] -> w304
                  tunnel: w303 -> [w318 _]
                  tunnel: w302 -> [w316 _]
                  frame False {
                    w313 = T24[] [enum."Manual All"] items=["No Action", "Reset Time", "Disable All", "Disable Lift", "Disable Arm", "Disable Claw Rotation", "Enable Lift", "Enable Arm", "Enable Claw Rotation", "Enable All", "Set Starting/Neutral", "Set Pickup/Exchange", "Set Switch", "Set Scale", "Set Climb", "Manual All", "Manual Arm", "Manual Lift", "Manual Claw Rotation", "Manual Off Arm", "Manual Off Lift", "Manual Off Claw Rotation", "Manual Off All", "Reset Stage Counter", "Increment Counter", "Manual Override", "Manual Override Off", "Netural Path - Arm First", "Neutral Path - Normal"] ("t")
                    w315 = ENUM_Overloard_State."Neutral - Moving" ("State")
                    n63 = case shown="8.." w318 {
                      tunnel: [ENUM_Overloard_Action."Increment Counter" ("Action") w326 w335 ENUM_Overloard_Action."Increment Counter" ("Action") w347 w356 w365 w383 ENUM_Overloard_Action."No Action" ("Action")] -> w317
                      tunnel: w316 -> [_ w330 w339 _ w351 w360 w369 w384 _]
                      tunnel: [FALSE FALSE FALSE FALSE FALSE FALSE FALSE FALSE TRUE] -> w311
                      tunnel: [ENUM_Overloard_Action."Disable All" ("Action") ENUM_Overloard_Action."Set Pickup/Exchange" ("Action") ENUM_Overloard_Action."Set Pickup/Exchange" ("Action") ENUM_Overloard_Action."Disable All" ("Action") ENUM_Overloard_Action."Set Starting/Neutral" ("Action") ENUM_Overloard_Action."Set Starting/Neutral" ("Action") ENUM_Overloard_Action."Set Starting/Neutral" ("Action") ENUM_Overloard_Action."Set Starting/Neutral" ("Action") ENUM_Overloard_Action."Set Starting/Neutral" ("Action")] -> w308
                      frame ..0 {
                      }
                      frame 1 {
                        n64 = Unbundle By Name(w330) -> ("Claw Rotation State"=w329:T22)
                        n65 = Equal?(x=w329, y=ENUM_SM_State."Position - Holding") -> (x = y?=w327:bool)
                        n66 = Select(t=ENUM_Overloard_Action."Increment Counter", s=w327, f=ENUM_Overloard_Action."Enable Claw Rotation" ("Action")) -> (s? t:f=w326:T24)
                      }
                      frame 2 {
                        n67 = Unbundle By Name(w339) -> ("Arm State"=w338:T23)
                        n68 = Equal?(x=w338, y=ENUM_SM_State."Position - Holding") -> (x = y?=w336:bool)
                        n69 = Select(t=ENUM_Overloard_Action."Increment Counter", s=w336, f=ENUM_Overloard_Action."Enable Arm" ("Action")) -> (s? t:f=w335:T24)
                      }
                      frame 3 {
                      }
                      frame 4 {
                        n70 = Unbundle By Name(w351) -> ("Arm State"=w350:T23)
                        n71 = Equal?(x=w350, y=ENUM_SM_State."Position - Holding") -> (x = y?=w348:bool)
                        n72 = Select(t=ENUM_Overloard_Action."Increment Counter", s=w348, f=ENUM_Overloard_Action."Enable Arm" ("Action")) -> (s? t:f=w347:T24)
                      }
                      frame 5 {
                        n73 = Unbundle By Name(w360) -> ("Claw Rotation State"=w359:T22)
                        n74 = Equal?(x=w359, y=ENUM_SM_State."Position - Holding") -> (x = y?=w357:bool)
                        n75 = Select(t=ENUM_Overloard_Action."Increment Counter", s=w357, f=ENUM_Overloard_Action."Enable Claw Rotation" ("Action")) -> (s? t:f=w356:T24)
                      }
                      frame 6 {
                        n76 = Unbundle By Name(w369) -> ("Lift State"=w368:T21)
                        n77 = Equal?(x=w368, y=ENUM_SM_State."Position - Holding") -> (x = y?=w366:bool)
                        n78 = Select(t=ENUM_Overloard_Action."Increment Counter", s=w366, f=ENUM_Overloard_Action."Enable Lift" ("Action")) -> (s? t:f=w365:T24)
                      }
                      frame 7 {
                        w380 = ENUM_SM_State."Position - Holding" ("y")
                        n79 = Unbundle By Name(w384) -> ("Lift State"=w379:T21, "Arm State"=w378:T23, "Claw Rotation State"=w377:T22)
                        n80 = Equal?(x=w380, y=w379) -> (x = y?=w376:bool)
                        n81 = Equal?(x=w380, y=w378) -> (x = y?=w375:bool)
                        n82 = Equal?(x=w380, y=w377) -> (x = y?=w373:bool)
                        n83 = And(x=w376, y=w375) -> (x .and. y?=w374:bool)
                        n84 = And(x=w374, y=w373) -> (x .and. y?=w372:bool)
                        n85 = Select(t=ENUM_Overloard_Action."Increment Counter", s=w372, f=ENUM_Overloard_Action."Enable All" ("Action")) -> (s? t:f=w383:T24)
                      }
                      frame 8.. {
                      }
                    }
                    n86 = Not(x=w311) -> (.not. x?=w310:bool)
                    n87 = Build Array(w317, w308, ENUM_Overloard_Action."Enable All" ("Action")) -> (w314:T24[])
                    n88 = Select(t=w315, s=w310, f=ENUM_Overloard_State."Neutral - Holding") -> ()  [unwired: 1 out]
                    n89 = Select(t=w313, s=w311, f=w314) -> ()  [unwired: 1 out]
                  }
                  frame True {
                    w388 = T24[] [] items=["No Action", "Reset Time", "Disable All", "Disable Lift", "Disable Arm", "Disable Claw Rotation", "Enable Lift", "Enable Arm", "Enable Claw Rotation", "Enable All", "Set Starting/Neutral", "Set Pickup/Exchange", "Set Switch", "Set Scale", "Set Climb", "Manual All", "Manual Arm", "Manual Lift", "Manual Claw Rotation", "Manual Off Arm", "Manual Off Lift", "Manual Off Claw Rotation", "Manual Off All", "Reset Stage Counter", "Increment Counter", "Manual Override", "Manual Override Off", "Netural Path - Arm First", "Neutral Path - Normal"] ("Actions")
                  }
                }
              }
              frame False {
                w390 = T24[] [enum."Set Starting/Neutral", enum."Manual Off All", enum."Reset Stage Counter", enum."Netural Path - Arm First"] items=["No Action", "Reset Time", "Disable All", "Disable Lift", "Disable Arm", "Disable Claw Rotation", "Enable Lift", "Enable Arm", "Enable Claw Rotation", "Enable All", "Set Starting/Neutral", "Set Pickup/Exchange", "Set Switch", "Set Scale", "Set Climb", "Manual All", "Manual Arm", "Manual Lift", "Manual Claw Rotation", "Manual Off Arm", "Manual Off Lift", "Manual Off Claw Rotation", "Manual Off All", "Reset Stage Counter", "Increment Counter", "Manual Override", "Manual Override Off", "Netural Path - Arm First", "Neutral Path - Normal"] ("Actions")
              }
            }
          }
        }
      }
      frame "Neutral - Holding" {
        w392 = T24[] [enum."Manual All"] items=["No Action", "Reset Time", "Disable All", "Disable Lift", "Disable Arm", "Disable Claw Rotation", "Enable Lift", "Enable Arm", "Enable Claw Rotation", "Enable All", "Set Starting/Neutral", "Set Pickup/Exchange", "Set Switch", "Set Scale", "Set Climb", "Manual All", "Manual Arm", "Manual Lift", "Manual Claw Rotation", "Manual Off Arm", "Manual Off Lift", "Manual Off Claw Rotation", "Manual Off All", "Reset Stage Counter", "Increment Counter", "Manual Override", "Manual Override Off", "Netural Path - Arm First", "Neutral Path - Normal"] ("Actions")
      }
      frame "Pickup - Moving" {
        # "Stage Counter\n-----------------\n0 - Setup\n1 - Moving Claw\n2 - Moving Arm\n3 - Moving Lift\n4 - All in Position\n5 - Position Held"
        n90 = Equal?(x=w401, y=w400) -> (x = y?=w399:bool)
        n91 = Unbundle By Name(w395) -> ("Stage Counter"=w396:i32)
        n92 = case shown="True" w399 {
          tunnel: [w405 ENUM_Overloard_State."Pickup - Moving" ("State")] -> w398
          tunnel: [w404 w463] -> w397
          tunnel: w396 -> [w403 _]
          tunnel: w395 -> [w402 _]
          frame True {
            n93 = Greater Or Equal?(x=w403, y=5) -> (x >= y?=w406:bool)
            n94 = case shown="False" w406 {
              tunnel: [w415 ENUM_Overloard_State."Pickup - Holding" ("State")] -> w405
              tunnel: [w414 w461] -> w404
              tunnel: w403 -> [w418 _]
              tunnel: w402 -> [w416 _]
              frame False {
                w413 = T24[] [enum."Manual All"] items=["No Action", "Reset Time", "Disable All", "Disable Lift", "Disable Arm", "Disable Claw Rotation", "Enable Lift", "Enable Arm", "Enable Claw Rotation", "Enable All", "Set Starting/Neutral", "Set Pickup/Exchange", "Set Switch", "Set Scale", "Set Climb", "Manual All", "Manual Arm", "Manual Lift", "Manual Claw Rotation", "Manual Off Arm", "Manual Off Lift", "Manual Off Claw Rotation", "Manual Off All", "Reset Stage Counter", "Increment Counter", "Manual Override", "Manual Override Off", "Netural Path - Arm First", "Neutral Path - Normal"] ("t")
                w415 = ENUM_Overloard_State."Pickup - Moving" ("State")
                n95 = case shown="2" w418 {
                  tunnel: [ENUM_Overloard_Action."Increment Counter" ("Action") w424 w432 w440 w457 ENUM_Overloard_Action."No Action" ("Action")] -> w417
                  tunnel: w416 -> [_ w428 w436 w444 w458 _]
                  tunnel: [FALSE FALSE FALSE FALSE FALSE TRUE] -> w411
                  frame ..0 {
                  }
                  frame 2 {
                    n96 = Unbundle By Name(w428) -> ("Arm State"=w427:T23)
                    n97 = Equal?(x=w427, y=ENUM_SM_State."Position - Holding") -> (x = y?=w425:bool)
                    n98 = Select(t=ENUM_Overloard_Action."Increment Counter", s=w425, f=ENUM_Overloard_Action."Manual Off Arm" ("Action")) -> (s? t:f=w424:T24)
                  }
                  frame 1 {
                    n99 = Unbundle By Name(w436) -> ("Claw Rotation State"=w435:T22)
                    n100 = Equal?(x=w435, y=ENUM_SM_State."Position - Holding") -> (x = y?=w433:bool)
                    n101 = Select(t=ENUM_Overloard_Action."Increment Counter", s=w433, f=ENUM_Overloard_Action."Manual Off Claw Rotation" ("Action")) -> (s? t:f=w432:T24)
                  }
                  frame 3 {
                    n102 = Unbundle By Name(w444) -> ("Lift State"=w443:T21)
                    n103 = Equal?(x=w443, y=ENUM_SM_State."Position - Holding") -> (x = y?=w441:bool)
                    n104 = Select(t=ENUM_Overloard_Action."Increment Counter", s=w441, f=ENUM_Overloard_Action."Manual Off Lift" ("Action")) -> (s? t:f=w440:T24)
                  }
                  frame 4 {
                    w454 = ENUM_SM_State."Position - Holding" ("y")
                    n105 = Unbundle By Name(w458) -> ("Lift State"=w453:T21, "Arm State"=w452:T23, "Claw Rotation State"=w451:T22)
                    n106 = Equal?(x=w454, y=w453) -> (x = y?=w450:bool)
                    n107 = Equal?(x=w454, y=w452) -> (x = y?=w449:bool)
                    n108 = Equal?(x=w454, y=w451) -> (x = y?=w447:bool)
                    n109 = And(x=w450, y=w449) -> (x .and. y?=w448:bool)
                    n110 = And(x=w448, y=w447) -> (x .and. y?=w446:bool)
                    n111 = Select(t=ENUM_Overloard_Action."Increment Counter", s=w446, f=ENUM_Overloard_Action."Manual Off All" ("Action")) -> (s? t:f=w457:T24)
                  }
                  frame 5.. {
                  }
                }
                n112 = Not(x=w411) -> (.not. x?=w410:bool)
                n113 = Build Array(w417, ENUM_Overloard_Action."Enable All" ("Action"), ENUM_Overloard_Action."Set Pickup/Exchange" ("Action")) -> (w414:T24[])
                n114 = Select(t=w415, s=w410, f=ENUM_Overloard_State."Pickup - Holding") -> ()  [unwired: 1 out]
                n115 = Select(t=w413, s=w411, f=w414) -> ()  [unwired: 1 out]
              }
              frame True {
                w461 = T24[] [] items=["No Action", "Reset Time", "Disable All", "Disable Lift", "Disable Arm", "Disable Claw Rotation", "Enable Lift", "Enable Arm", "Enable Claw Rotation", "Enable All", "Set Starting/Neutral", "Set Pickup/Exchange", "Set Switch", "Set Scale", "Set Climb", "Manual All", "Manual Arm", "Manual Lift", "Manual Claw Rotation", "Manual Off Arm", "Manual Off Lift", "Manual Off Claw Rotation", "Manual Off All", "Reset Stage Counter", "Increment Counter", "Manual Override", "Manual Override Off", "Netural Path - Arm First", "Neutral Path - Normal"] ("Actions")
              }
            }
          }
          frame False {
            w463 = T24[] [enum."Set Pickup/Exchange", enum."Manual All", enum."Reset Stage Counter", enum."Neutral Path - Normal"] items=["No Action", "Reset Time", "Disable All", "Disable Lift", "Disable Arm", "Disable Claw Rotation", "Enable Lift", "Enable Arm", "Enable Claw Rotation", "Enable All", "Set Starting/Neutral", "Set Pickup/Exchange", "Set Switch", "Set Scale", "Set Climb", "Manual All", "Manual Arm", "Manual Lift", "Manual Claw Rotation", "Manual Off Arm", "Manual Off Lift", "Manual Off Claw Rotation", "Manual Off All", "Reset Stage Counter", "Increment Counter", "Manual Override", "Manual Override Off", "Netural Path - Arm First", "Neutral Path - Normal"] ("Actions")
          }
        }
      }
      frame "Pickup - Holding" {
        w465 = T24[] [enum."Manual All"] items=["No Action", "Reset Time", "Disable All", "Disable Lift", "Disable Arm", "Disable Claw Rotation", "Enable Lift", "Enable Arm", "Enable Claw Rotation", "Enable All", "Set Starting/Neutral", "Set Pickup/Exchange", "Set Switch", "Set Scale", "Set Climb", "Manual All", "Manual Arm", "Manual Lift", "Manual Claw Rotation", "Manual Off Arm", "Manual Off Lift", "Manual Off Claw Rotation", "Manual Off All", "Reset Stage Counter", "Increment Counter", "Manual Override", "Manual Override Off", "Netural Path - Arm First", "Neutral Path - Normal"] ("Actions")
      }
      frame "Switch - Moving" {
        # "Stage Counter\n-----------------\n0 - Setup\n1 - Moving Arm\n2 - Moving Claw\n3 - Moving Lift\n4 - All in Position\n5 - Position Held"
        n116 = Equal?(x=w474, y=w473) -> (x = y?=w472:bool)
        n117 = Unbundle By Name(w468) -> ("Stage Counter"=w469:i32)
        n118 = case shown="False" w472 {
          tunnel: [w478 ENUM_Overloard_State."Switch - Moving" ("State")] -> w471
          tunnel: [w477 w536] -> w470
          tunnel: w469 -> [w476 _]
          tunnel: w468 -> [w475 _]
          frame True {
            n119 = Greater Or Equal?(x=w476, y=5) -> (x >= y?=w479:bool)
            n120 = case shown="False" w479 {
              tunnel: [w487 ENUM_Overloard_State."Switch - Holding" ("State")] -> w478
              tunnel: [w486 w534] -> w477
              tunnel: w476 -> [w491 _]
              tunnel: w475 -> [w488 _]
              frame False {
                w485 = T24[] [enum."Manual All"] items=["No Action", "Reset Time", "Disable All", "Disable Lift", "Disable Arm", "Disable Claw Rotation", "Enable Lift", "Enable Arm", "Enable Claw Rotation", "Enable All", "Set Starting/Neutral", "Set Pickup/Exchange", "Set Switch", "Set Scale", "Set Climb", "Manual All", "Manual Arm", "Manual Lift", "Manual Claw Rotation", "Manual Off Arm", "Manual Off Lift", "Manual Off Claw Rotation", "Manual Off All", "Reset Stage Counter", "Increment Counter", "Manual Override", "Manual Override Off", "Netural Path - Arm First", "Neutral Path - Normal"] ("t")
                w487 = ENUM_Overloard_State."Switch - Moving" ("State")
                n121 = case shown="5.." w491 {
                  tunnel: [ENUM_Overloard_Action."Increment Counter" ("Action") w497 w505 w513 w530 ENUM_Overloard_Action."No Action" ("Action")] -> w490
                  tunnel: w488 -> [_ w501 w509 w517 w531 _]
                  tunnel: [FALSE FALSE FALSE FALSE FALSE TRUE] -> w483
                  frame ..0 {
                  }
                  frame 1 {
                    n122 = Unbundle By Name(w501) -> ("Arm State"=w500:T23)
                    n123 = Equal?(x=w500, y=ENUM_SM_State."Position - Holding") -> (x = y?=w498:bool)
                    n124 = Select(t=ENUM_Overloard_Action."Increment Counter", s=w498, f=ENUM_Overloard_Action."Manual Off Arm" ("Action")) -> (s? t:f=w497:T24)
                  }
                  frame 2 {
                    n125 = Unbundle By Name(w509) -> ("Claw Rotation State"=w508:T22)
                    n126 = Equal?(x=w508, y=ENUM_SM_State."Position - Holding") -> (x = y?=w506:bool)
                    n127 = Select(t=ENUM_Overloard_Action."Increment Counter", s=w506, f=ENUM_Overloard_Action."Manual Off Claw Rotation" ("Action")) -> (s? t:f=w505:T24)
                  }
                  frame 3 {
                    n128 = Unbundle By Name(w517) -> ("Lift State"=w516:T21)
                    n129 = Equal?(x=w516, y=ENUM_SM_State."Position - Holding") -> (x = y?=w514:bool)
                    n130 = Select(t=ENUM_Overloard_Action."Increment Counter", s=w514, f=ENUM_Overloard_Action."Manual Off Lift" ("Action")) -> (s? t:f=w513:T24)
                  }
                  frame 4 {
                    w527 = ENUM_SM_State."Position - Holding" ("y")
                    n131 = Unbundle By Name(w531) -> ("Lift State"=w526:T21, "Arm State"=w525:T23, "Claw Rotation State"=w524:T22)
                    n132 = Equal?(x=w527, y=w526) -> (x = y?=w523:bool)
                    n133 = Equal?(x=w527, y=w525) -> (x = y?=w522:bool)
                    n134 = Equal?(x=w527, y=w524) -> (x = y?=w520:bool)
                    n135 = And(x=w523, y=w522) -> (x .and. y?=w521:bool)
                    n136 = And(x=w521, y=w520) -> (x .and. y?=w519:bool)
                    n137 = Select(t=ENUM_Overloard_Action."Increment Counter", s=w519, f=ENUM_Overloard_Action."Manual Off All" ("Action")) -> (s? t:f=w530:T24)
                  }
                  frame 5.. {
                  }
                }
                n138 = Not(x=w483) -> (.not. x?=w482:bool)
                n139 = Build Array(w490, ENUM_Overloard_Action."Set Switch" ("Action"), ENUM_Overloard_Action."Enable All" ("element")) -> (w486:T24[])
                n140 = Select(t=w487, s=w482, f=ENUM_Overloard_State."Switch - Holding") -> ()  [unwired: 1 out]
                n141 = Select(t=w485, s=w483, f=w486) -> ()  [unwired: 1 out]
              }
              frame True {
                w534 = T24[] [] items=["No Action", "Reset Time", "Disable All", "Disable Lift", "Disable Arm", "Disable Claw Rotation", "Enable Lift", "Enable Arm", "Enable Claw Rotation", "Enable All", "Set Starting/Neutral", "Set Pickup/Exchange", "Set Switch", "Set Scale", "Set Climb", "Manual All", "Manual Arm", "Manual Lift", "Manual Claw Rotation", "Manual Off Arm", "Manual Off Lift", "Manual Off Claw Rotation", "Manual Off All", "Reset Stage Counter", "Increment Counter", "Manual Override", "Manual Override Off", "Netural Path - Arm First", "Neutral Path - Normal"] ("Actions")
              }
            }
          }
          frame False {
            w536 = T24[] [enum."Set Switch", enum."Manual All", enum."Reset Stage Counter", enum."Neutral Path - Normal"] items=["No Action", "Reset Time", "Disable All", "Disable Lift", "Disable Arm", "Disable Claw Rotation", "Enable Lift", "Enable Arm", "Enable Claw Rotation", "Enable All", "Set Starting/Neutral", "Set Pickup/Exchange", "Set Switch", "Set Scale", "Set Climb", "Manual All", "Manual Arm", "Manual Lift", "Manual Claw Rotation", "Manual Off Arm", "Manual Off Lift", "Manual Off Claw Rotation", "Manual Off All", "Reset Stage Counter", "Increment Counter", "Manual Override", "Manual Override Off", "Netural Path - Arm First", "Neutral Path - Normal"] ("Actions")
          }
        }
      }
      frame "Switch - Holding" {
        w538 = T24[] [enum."Manual All"] items=["No Action", "Reset Time", "Disable All", "Disable Lift", "Disable Arm", "Disable Claw Rotation", "Enable Lift", "Enable Arm", "Enable Claw Rotation", "Enable All", "Set Starting/Neutral", "Set Pickup/Exchange", "Set Switch", "Set Scale", "Set Climb", "Manual All", "Manual Arm", "Manual Lift", "Manual Claw Rotation", "Manual Off Arm", "Manual Off Lift", "Manual Off Claw Rotation", "Manual Off All", "Reset Stage Counter", "Increment Counter", "Manual Override", "Manual Override Off", "Netural Path - Arm First", "Neutral Path - Normal"] ("Actions")
      }
      frame "Scale - Moving" {
        # "Stage Counter\n-----------------\n0 - Setup\n1 - Set Lift - Neutral\n2 - Set Arm - Neutral\n3 - Set Claw - Neutral\n4 - Reset for Scale\n5 - Moving Lift\n6 - Moving Claw\n7 - Moving Arm\n8 - All in Position\n9 - Position Held"
        n142 = Equal?(x=w547, y=w546) -> (x = y?=w545:bool)
        n143 = Unbundle By Name(w541) -> ("Stage Counter"=w542:i32)
        n144 = case shown="False" w545 {
          tunnel: [w551 ENUM_Overloard_State."Scale - Moving" ("State")] -> w544
          tunnel: [w550 w644] -> w543
          tunnel: w542 -> [w549 _]
          tunnel: w541 -> [w548 _]
          frame True {
            n145 = Greater Or Equal?(x=w549, y=9) -> (x >= y?=w552:bool)
            n146 = case shown="False" w552 {
              tunnel: [w560 ENUM_Overloard_State."Scale - Holding" ("State")] -> w551
              tunnel: [w559 w642] -> w550
              tunnel: w549 -> [w563 _]
              tunnel: w548 -> [w561 _]
              frame False {
                w558 = T24[] [enum."Manual All"] items=["No Action", "Reset Time", "Disable All", "Disable Lift", "Disable Arm", "Disable Claw Rotation", "Enable Lift", "Enable Arm", "Enable Claw Rotation", "Enable All", "Set Starting/Neutral", "Set Pickup/Exchange", "Set Switch", "Set Scale", "Set Climb", "Manual All", "Manual Arm", "Manual Lift", "Manual Claw Rotation", "Manual Off Arm", "Manual Off Lift", "Manual Off Claw Rotation", "Manual Off All", "Reset Stage Counter", "Increment Counter", "Manual Override", "Manual Override Off", "Netural Path - Arm First", "Neutral Path - Normal"] ("t")
                w560 = ENUM_Overloard_State."Scale - Moving" ("State")
                n147 = case shown="1" w563 {
                  tunnel: [ENUM_Overloard_Action."Increment Counter" ("Action") w571 w580 w589 ENUM_Overloard_Action."Increment Counter" ("Action") w601 w610 w619 w637 ENUM_Overloard_Action."No Action" ("Action")] -> w562
                  tunnel: w561 -> [_ w575 w584 w593 _ w605 w614 w623 w638 _]
                  tunnel: [FALSE FALSE FALSE FALSE FALSE FALSE FALSE FALSE FALSE TRUE] -> w556
                  tunnel: [ENUM_Overloard_Action."Set Starting/Neutral" ("Action") ENUM_Overloard_Action."Set Starting/Neutral" ("Action") ENUM_Overloard_Action."Set Starting/Neutral" ("Action") ENUM_Overloard_Action."Set Starting/Neutral" ("Action") ENUM_Overloard_Action."Manual All" ("Action") ENUM_Overloard_Action."Set Scale" ("Action") ENUM_Overloard_Action."Set Scale" ("Action") ENUM_Overloard_Action."Set Scale" ("Action") ENUM_Overloard_Action."Set Scale" ("Action") ENUM_Overloard_Action."Set Scale" ("Action")] -> w554
                  frame ..0 {
                  }
                  frame 1 {
                    n148 = Unbundle By Name(w575) -> ("Lift State"=w574:T21)
                    n149 = Equal?(x=w574, y=ENUM_SM_State."Position - Holding") -> (x = y?=w572:bool)
                    n150 = Select(t=ENUM_Overloard_Action."Increment Counter", s=w572, f=ENUM_Overloard_Action."Manual Off Lift" ("Action")) -> (s? t:f=w571:T24)
                  }
                  frame 2 {
                    n151 = Unbundle By Name(w584) -> ("Claw Rotation State"=w583:T22)
                    n152 = Equal?(x=w583, y=ENUM_SM_State."Position - Holding") -> (x = y?=w581:bool)
                    n153 = Select(t=ENUM_Overloard_Action."Increment Counter", s=w581, f=ENUM_Overloard_Action."Manual Off Claw Rotation" ("Action")) -> (s? t:f=w580:T24)
                  }
                  frame 3 {
                    n154 = Unbundle By Name(w593) -> ("Arm State"=w592:T23)
                    n155 = Equal?(x=w592, y=ENUM_SM_State."Position - Holding") -> (x = y?=w590:bool)
                    n156 = Select(t=ENUM_Overloard_Action."Increment Counter", s=w590, f=ENUM_Overloard_Action."Manual Off Arm" ("Action")) -> (s? t:f=w589:T24)
                  }
                  frame 4 {
                  }
                  frame 5 {
                    n157 = Unbundle By Name(w605) -> ("Lift State"=w604:T21)
                    n158 = Equal?(x=w604, y=ENUM_SM_State."Position - Holding") -> (x = y?=w602:bool)
                    n159 = Select(t=ENUM_Overloard_Action."Increment Counter", s=w602, f=ENUM_Overloard_Action."Manual Off Lift" ("Action")) -> (s? t:f=w601:T24)
                  }
                  frame 6 {
                    n160 = Unbundle By Name(w614) -> ("Claw Rotation State"=w613:T22)
                    n161 = Equal?(x=w613, y=ENUM_SM_State."Position - Holding") -> (x = y?=w611:bool)
                    n162 = Select(t=ENUM_Overloard_Action."Increment Counter", s=w611, f=ENUM_Overloard_Action."Manual Off Claw Rotation" ("Action")) -> (s? t:f=w610:T24)
                  }
                  frame 7 {
                    n163 = Unbundle By Name(w623) -> ("Arm State"=w622:T23)
                    n164 = Equal?(x=w622, y=ENUM_SM_State."Position - Holding") -> (x = y?=w620:bool)
                    n165 = Select(t=ENUM_Overloard_Action."Increment Counter", s=w620, f=ENUM_Overloard_Action."Manual Off Arm" ("Action")) -> (s? t:f=w619:T24)
                  }
                  frame 8 {
                    w634 = ENUM_SM_State."Position - Holding" ("y")
                    n166 = Unbundle By Name(w638) -> ("Lift State"=w633:T21, "Arm State"=w632:T23, "Claw Rotation State"=w631:T22)
                    n167 = Equal?(x=w634, y=w633) -> (x = y?=w630:bool)
                    n168 = Equal?(x=w634, y=w632) -> (x = y?=w629:bool)
                    n169 = Equal?(x=w634, y=w631) -> (x = y?=w627:bool)
                    n170 = And(x=w630, y=w629) -> (x .and. y?=w628:bool)
                    n171 = And(x=w628, y=w627) -> (x .and. y?=w626:bool)
                    n172 = Select(t=ENUM_Overloard_Action."Increment Counter", s=w626, f=ENUM_Overloard_Action."Manual Off All" ("Action")) -> (s? t:f=w637:T24)
                  }
                  frame 9.. {
                  }
                }
                n173 = Not(x=w556) -> (.not. x?=w555:bool)
                n174 = Build Array(w562, w554) -> (w559:T24[])
                n175 = Select(t=w560, s=w555, f=ENUM_Overloard_State."Scale - Holding") -> ()  [unwired: 1 out]
                n176 = Select(t=w558, s=w556, f=w559) -> ()  [unwired: 1 out]
              }
              frame True {
                w642 = T24[] [] items=["No Action", "Reset Time", "Disable All", "Disable Lift", "Disable Arm", "Disable Claw Rotation", "Enable Lift", "Enable Arm", "Enable Claw Rotation", "Enable All", "Set Starting/Neutral", "Set Pickup/Exchange", "Set Switch", "Set Scale", "Set Climb", "Manual All", "Manual Arm", "Manual Lift", "Manual Claw Rotation", "Manual Off Arm", "Manual Off Lift", "Manual Off Claw Rotation", "Manual Off All", "Reset Stage Counter", "Increment Counter", "Manual Override", "Manual Override Off", "Netural Path - Arm First", "Neutral Path - Normal"] ("Actions")
              }
            }
          }
          frame False {
            w644 = T24[] [enum."Set Scale", enum."Manual All", enum."Reset Stage Counter", enum."Neutral Path - Normal"] items=["No Action", "Reset Time", "Disable All", "Disable Lift", "Disable Arm", "Disable Claw Rotation", "Enable Lift", "Enable Arm", "Enable Claw Rotation", "Enable All", "Set Starting/Neutral", "Set Pickup/Exchange", "Set Switch", "Set Scale", "Set Climb", "Manual All", "Manual Arm", "Manual Lift", "Manual Claw Rotation", "Manual Off Arm", "Manual Off Lift", "Manual Off Claw Rotation", "Manual Off All", "Reset Stage Counter", "Increment Counter", "Manual Override", "Manual Override Off", "Netural Path - Arm First", "Neutral Path - Normal"] ("Actions")
          }
        }
      }
      frame "Scale - Holding" {
        w646 = T24[] [enum."Manual All"] items=["No Action", "Reset Time", "Disable All", "Disable Lift", "Disable Arm", "Disable Claw Rotation", "Enable Lift", "Enable Arm", "Enable Claw Rotation", "Enable All", "Set Starting/Neutral", "Set Pickup/Exchange", "Set Switch", "Set Scale", "Set Climb", "Manual All", "Manual Arm", "Manual Lift", "Manual Claw Rotation", "Manual Off Arm", "Manual Off Lift", "Manual Off Claw Rotation", "Manual Off All", "Reset Stage Counter", "Increment Counter", "Manual Override", "Manual Override Off", "Netural Path - Arm First", "Neutral Path - Normal"] ("Actions")
      }
      frame "Climb - Moving" {
        # "Stage Counter\n-----------------\n0 - Setup\n1 - Moving Lift\n2 - Moving Claw\n3 - Moving Arm\n4 - All in Position\n5 - Position Held"
        n177 = Equal?(x=w655, y=w654) -> (x = y?=w653:bool)
        n178 = Unbundle By Name(w649) -> ("Stage Counter"=w650:i32)
        n179 = case shown="True" w653 {
          tunnel: [w659 ENUM_Overloard_State."Climb - Moving" ("State")] -> w652
          tunnel: [w658 w716] -> w651
          tunnel: w650 -> [w657 _]
          tunnel: w649 -> [w656 _]
          frame True {
            n180 = Greater Or Equal?(x=w657, y=5) -> (x >= y?=w660:bool)
            n181 = case shown="False" w660 {
              tunnel: [w667 ENUM_Overloard_State."Climb - Holding" ("State")] -> w659
              tunnel: [w666 w714] -> w658
              tunnel: w657 -> [w671 _]
              tunnel: w656 -> [w668 _]
              frame False {
                w665 = T24[] [enum."Manual All"] items=["No Action", "Reset Time", "Disable All", "Disable Lift", "Disable Arm", "Disable Claw Rotation", "Enable Lift", "Enable Arm", "Enable Claw Rotation", "Enable All", "Set Starting/Neutral", "Set Pickup/Exchange", "Set Switch", "Set Scale", "Set Climb", "Manual All", "Manual Arm", "Manual Lift", "Manual Claw Rotation", "Manual Off Arm", "Manual Off Lift", "Manual Off Claw Rotation", "Manual Off All", "Reset Stage Counter", "Increment Counter", "Manual Override", "Manual Override Off", "Netural Path - Arm First", "Neutral Path - Normal"] ("t")
                w667 = ENUM_Overloard_State."Climb - Moving" ("State")
                n182 = case shown="1" w671 {
                  tunnel: [ENUM_Overloard_Action."Increment Counter" ("Action") w677 w685 w693 w710 ENUM_Overloard_Action."No Action" ("Action")] -> w670
                  tunnel: w668 -> [_ w681 w689 w697 w711 _]
                  tunnel: [FALSE FALSE FALSE FALSE FALSE TRUE] -> w663
                  frame ..0 {
                  }
                  frame 1 {
                    n183 = Unbundle By Name(w681) -> ("Lift State"=w680:T21)
                    n184 = Equal?(x=w680, y=ENUM_SM_State."Position - Holding") -> (x = y?=w678:bool)
                    n185 = Select(t=ENUM_Overloard_Action."Increment Counter", s=w678, f=ENUM_Overloard_Action."Manual Off Lift" ("Action")) -> (s? t:f=w677:T24)
                  }
                  frame 2 {
                    n186 = Unbundle By Name(w689) -> ("Claw Rotation State"=w688:T22)
                    n187 = Equal?(x=w688, y=ENUM_SM_State."Position - Holding") -> (x = y?=w686:bool)
                    n188 = Select(t=ENUM_Overloard_Action."Increment Counter", s=w686, f=ENUM_Overloard_Action."Manual Off Claw Rotation" ("Action")) -> (s? t:f=w685:T24)
                  }
                  frame 3 {
                    n189 = Unbundle By Name(w697) -> ("Arm State"=w696:T23)
                    n190 = Equal?(x=w696, y=ENUM_SM_State."Position - Holding") -> (x = y?=w694:bool)
                    n191 = Select(t=ENUM_Overloard_Action."Increment Counter", s=w694, f=ENUM_Overloard_Action."Manual Off Arm" ("Action")) -> (s? t:f=w693:T24)
                  }
                  frame 4 {
                    w707 = ENUM_SM_State."Position - Holding" ("y")
                    n192 = Unbundle By Name(w711) -> ("Lift State"=w706:T21, "Arm State"=w705:T23, "Claw Rotation State"=w704:T22)
                    n193 = Equal?(x=w707, y=w706) -> (x = y?=w703:bool)
                    n194 = Equal?(x=w707, y=w705) -> (x = y?=w702:bool)
                    n195 = Equal?(x=w707, y=w704) -> (x = y?=w700:bool)
                    n196 = And(x=w703, y=w702) -> (x .and. y?=w701:bool)
                    n197 = And(x=w701, y=w700) -> (x .and. y?=w699:bool)
                    n198 = Select(t=ENUM_Overloard_Action."Increment Counter", s=w699, f=ENUM_Overloard_Action."Manual Off All" ("Action")) -> (s? t:f=w710:T24)
                  }
                  frame 5.. {
                  }
                }
                n199 = Not(x=w663) -> (.not. x?=w662:bool)
                n200 = Build Array(w670, ENUM_Overloard_Action."Set Climb" ("Action")) -> (w666:T24[])
                n201 = Select(t=w667, s=w662, f=ENUM_Overloard_State."Climb - Holding") -> ()  [unwired: 1 out]
                n202 = Select(t=w665, s=w663, f=w666) -> ()  [unwired: 1 out]
              }
              frame True {
                w714 = T24[] [] items=["No Action", "Reset Time", "Disable All", "Disable Lift", "Disable Arm", "Disable Claw Rotation", "Enable Lift", "Enable Arm", "Enable Claw Rotation", "Enable All", "Set Starting/Neutral", "Set Pickup/Exchange", "Set Switch", "Set Scale", "Set Climb", "Manual All", "Manual Arm", "Manual Lift", "Manual Claw Rotation", "Manual Off Arm", "Manual Off Lift", "Manual Off Claw Rotation", "Manual Off All", "Reset Stage Counter", "Increment Counter", "Manual Override", "Manual Override Off", "Netural Path - Arm First", "Neutral Path - Normal"] ("Actions")
              }
            }
          }
          frame False {
            w716 = T24[] [enum."Set Climb", enum."Manual All", enum."Reset Stage Counter", enum."Neutral Path - Normal"] items=["No Action", "Reset Time", "Disable All", "Disable Lift", "Disable Arm", "Disable Claw Rotation", "Enable Lift", "Enable Arm", "Enable Claw Rotation", "Enable All", "Set Starting/Neutral", "Set Pickup/Exchange", "Set Switch", "Set Scale", "Set Climb", "Manual All", "Manual Arm", "Manual Lift", "Manual Claw Rotation", "Manual Off Arm", "Manual Off Lift", "Manual Off Claw Rotation", "Manual Off All", "Reset Stage Counter", "Increment Counter", "Manual Override", "Manual Override Off", "Netural Path - Arm First", "Neutral Path - Normal"] ("Actions")
          }
        }
      }
      frame "Climb - Holding" {
        w718 = T24[] [enum."Manual All"] items=["No Action", "Reset Time", "Disable All", "Disable Lift", "Disable Arm", "Disable Claw Rotation", "Enable Lift", "Enable Arm", "Enable Claw Rotation", "Enable All", "Set Starting/Neutral", "Set Pickup/Exchange", "Set Switch", "Set Scale", "Set Climb", "Manual All", "Manual Arm", "Manual Lift", "Manual Claw Rotation", "Manual Off Arm", "Manual Off Lift", "Manual Off Claw Rotation", "Manual Off All", "Reset Stage Counter", "Increment Counter", "Manual Override", "Manual Override Off", "Netural Path - Arm First", "Neutral Path - Normal"] ("Actions")
      }
      frame "F_Manual" {
        w721 = T24[] [enum."Manual Override"] items=["No Action", "Reset Time", "Disable All", "Disable Lift", "Disable Arm", "Disable Claw Rotation", "Enable Lift", "Enable Arm", "Enable Claw Rotation", "Enable All", "Set Starting/Neutral", "Set Pickup/Exchange", "Set Switch", "Set Scale", "Set Climb", "Manual All", "Manual Arm", "Manual Lift", "Manual Claw Rotation", "Manual Off Arm", "Manual Off Lift", "Manual Off Claw Rotation", "Manual Off All", "Reset Stage Counter", "Increment Counter", "Manual Override", "Manual Override Off", "Netural Path - Arm First", "Neutral Path - Normal"] ("Actions")
      }
      frame "Manual" {
        n203 = Unbundle By Name(w729) -> ("Rotation CMD.Rotation Positon"=w728:T9, "Previous Rotation CMD.Rotation Positon"=w727:T9)
        n204 = Equal?(x=w728, y=w727) -> (x = y?=w726:bool)
        n205 = case shown="False" w726 {
          tunnel: [w731 w733] -> w725
          tunnel: [ENUM_Overloard_State."Manual" ("State") ENUM_Overloard_State."Idle" ("State")] -> w724
          frame True {
            w731 = T24[] [enum."Manual All", enum."Manual Override Off", enum."Enable All"] items=["No Action", "Reset Time", "Disable All", "Disable Lift", "Disable Arm", "Disable Claw Rotation", "Enable Lift", "Enable Arm", "Enable Claw Rotation", "Enable All", "Set Starting/Neutral", "Set Pickup/Exchange", "Set Switch", "Set Scale", "Set Climb", "Manual All", "Manual Arm", "Manual Lift", "Manual Claw Rotation", "Manual Off Arm", "Manual Off Lift", "Manual Off Claw Rotation", "Manual Off All", "Reset Stage Counter", "Increment Counter", "Manual Override", "Manual Override Off", "Netural Path - Arm First", "Neutral Path - Normal"] ("Actions")
          }
          frame False {
            w733 = T24[] [enum."Manual Off All", enum."Manual Override Off"] items=["No Action", "Reset Time", "Disable All", "Disable Lift", "Disable Arm", "Disable Claw Rotation", "Enable Lift", "Enable Arm", "Enable Claw Rotation", "Enable All", "Set Starting/Neutral", "Set Pickup/Exchange", "Set Switch", "Set Scale", "Set Climb", "Manual All", "Manual Arm", "Manual Lift", "Manual Claw Rotation", "Manual Off Arm", "Manual Off Lift", "Manual Off Claw Rotation", "Manual Off All", "Reset Stage Counter", "Increment Counter", "Manual Override", "Manual Override Off", "Netural Path - Arm First", "Neutral Path - Normal"] ("Actions")
          }
        }
      }
      frame "Shutdown" {
        w735 = T24[] [enum."Disable All"] items=["No Action", "Reset Time", "Disable All", "Disable Lift", "Disable Arm", "Disable Claw Rotation", "Enable Lift", "Enable Arm", "Enable Claw Rotation", "Enable All", "Set Starting/Neutral", "Set Pickup/Exchange", "Set Switch", "Set Scale", "Set Climb", "Manual All", "Manual Arm", "Manual Lift", "Manual Claw Rotation", "Manual Off Arm", "Manual Off Lift", "Manual Off Claw Rotation", "Manual Off All", "Reset Stage Counter", "Increment Counter", "Manual Override", "Manual Override Off", "Netural Path - Arm First", "Neutral Path - Normal"] ("Actions")
      }
    }
    n206 = Bundle By Name(cluster=w27, "Previous State"=w54, "State"=w37) -> (w59:T25)
    n207 = for {
      shift-right: [w63] -> w53
      shift-left: w59 -> [w62]
      tunnel: w38 -> [w61] mode=indexing
      n208 = case shown="\"Enable Claw Rotation\"" w61 {
        tunnel: w62 -> [w64 w67 w72 w75 w78 w81 w84 w87 w90 w95 w100 w105 w110 w115 w120 w124 w130 w134 w138 w142 w146 w150 w156 w163 w165 w170 w173 w176 w179]
        tunnel: [w64 w66 w71 w74 w77 w80 w83 w86 w89 w94 w99 w104 w109 w114 w119 w128 w132 w136 w140 w144 w148 w152 w160 w162 w164 w169 w172 w175 w178] -> w63
        frame "No Action" {
        }
        frame "Reset Time" {
          # "Reset timer by taking the current time\nand making it the start time\n\nLater when the current time is \nsubtracted from the start time\nyou will get the elapsed time in \nseconds"
          n209 = Unbundle By Name(w67) -> ("Current Time"=w65:timestamp)
          n210 = Bundle By Name(cluster=w67, "Start Time"=w65) -> (w66:T25)
        }
        frame "Disable All" {
          n211 = Bundle By Name(cluster=w72, "Arm CMD.Enable System"=FALSE, "Claw Rotation CMD.Enable System"=FALSE, "Lift CMD.Enable System"=FALSE) -> (w71:T25)
        }
        frame "Disable Lift" {
          n212 = Bundle By Name(cluster=w75, "Lift CMD.Enable System"=FALSE) -> (w74:T25)
        }
        frame "Disable Arm" {
          n213 = Bundle By Name(cluster=w78, "Arm CMD.Enable System"=FALSE ("Lift CMD.Enable System")) -> (w77:T25)
        }
        frame "Disable Claw Rotation" {
          n214 = Bundle By Name(cluster=w81, "Claw Rotation CMD.Enable System"=FALSE ("Lift CMD.Enable System")) -> (w80:T25)
        }
        frame "Enable Lift" {
          n215 = Bundle By Name(cluster=w84, "Lift CMD.Enable System"=TRUE) -> (w83:T25)
        }
        frame "Enable Arm" {
          n216 = Bundle By Name(cluster=w87, "Arm CMD.Enable System"=TRUE ("Lift CMD.Enable System")) -> (w86:T25)
        }
        frame "Enable Claw Rotation" {
          n217 = Bundle By Name(cluster=w90, "Claw Rotation CMD.Enable System"=TRUE ("Lift CMD.Enable System")) -> (w89:T25)
        }
        frame "Enable All" {
          n218 = Bundle By Name(cluster=w95, "Arm CMD.Enable System"=TRUE, "Claw Rotation CMD.Enable System"=TRUE, "Lift CMD.Enable System"=TRUE) -> (w94:T25)
        }
        frame "Set Starting/Neutral" {
          n219 = Bundle By Name(cluster=w100, "Arm CMD.Rotate Position"=ENUM_SM_Rotate_Positions."Neutral: 3230", "Claw Rotation CMD.Rotate Position"=ENUM_SM_Rotate_Positions."Neutral: -500", "Lift CMD.Rotate Position"=ENUM_SM_Rotate_Positions."Neutral: 0") -> (w99:T25)
        }
        frame "Set Pickup/Exchange" {
          n220 = Bundle By Name(cluster=w105, "Arm CMD.Rotate Position"=ENUM_SM_Rotate_Positions."Pickup: 0", "Claw Rotation CMD.Rotate Position"=ENUM_SM_Rotate_Positions."Pickup: -700", "Lift CMD.Rotate Position"=ENUM_SM_Rotate_Positions."Pickup: 0") -> (w104:T25)
        }
        frame "Set Switch" {
          n221 = Bundle By Name(cluster=w110, "Arm CMD.Rotate Position"=ENUM_SM_Rotate_Positions."Switch: 2100", "Claw Rotation CMD.Rotate Position"=ENUM_SM_Rotate_Positions."Switch: -700", "Lift CMD.Rotate Position"=ENUM_SM_Rotate_Positions."Switch: 0") -> (w109:T25)
        }
        frame "Set Scale" {
          n222 = Bundle By Name(cluster=w115, "Arm CMD.Rotate Position"=ENUM_SM_Rotate_Positions."Scale: 3700", "Claw Rotation CMD.Rotate Position"=ENUM_SM_Rotate_Positions."Scale: 0", "Lift CMD.Rotate Position"=ENUM_SM_Rotate_Positions."Scale:  117000") -> (w114:T25)
        }
        frame "Set Climb" {
          n223 = Bundle By Name(cluster=w120, "Arm CMD.Rotate Position"=ENUM_SM_Rotate_Positions."Climb: 0", "Claw Rotation CMD.Rotate Position"=ENUM_SM_Rotate_Positions."Climb: 0", "Lift CMD.Rotate Position"=ENUM_SM_Rotate_Positions."Climb: 0") -> (w119:T25)
        }
        frame "Manual All" {
          n224 = Unbundle By Name(w124) -> ("Rotation CMD.Arm Value"=w121:dbl, "Rotation CMD.Claw Rotation Value"=w122:dbl, "Rotation CMD.Lift Value"=w123:dbl)
          n225 = Bundle By Name(cluster=w124, "Arm CMD.Manual Mode"=TRUE, "Claw Rotation CMD.Manual Mode"=TRUE, "Lift CMD.Manual Mode"=TRUE, "Arm CMD.Manual Velocity"=w121, "Claw Rotation CMD.Manual Velocity"=w122, "Lift CMD.Manual Velocity"=w123) -> (w128:T25)
        }
        frame "Manual Arm" {
          n226 = Unbundle By Name(w130) -> ("Rotation CMD.Arm Value"=w129:dbl)
          n227 = Bundle By Name(cluster=w130, "Arm CMD.Manual Mode"=TRUE, "Arm CMD.Manual Velocity"=w129) -> (w132:T25)
        }
        frame "Manual Lift" {
          n228 = Unbundle By Name(w134) -> ("Rotation CMD.Lift Value"=w133:dbl)
          n229 = Bundle By Name(cluster=w134, "Lift CMD.Manual Mode"=TRUE ("Arm CMD.Manual Mode"), "Lift CMD.Manual Velocity"=w133) -> (w136:T25)
        }
        frame "Manual Claw Rotation" {
          n230 = Unbundle By Name(w138) -> ("Rotation CMD.Claw Rotation Value"=w137:dbl)
          n231 = Bundle By Name(cluster=w138, "Claw Rotation CMD.Manual Mode"=TRUE ("Arm CMD.Manual Mode"), "Claw Rotation CMD.Manual Velocity"=w137) -> (w140:T25)
        }
        frame "Manual Off Arm" {
          n232 = Unbundle By Name(w142) -> ("Rotation CMD.Arm Value"=w141:dbl)
          n233 = Bundle By Name(cluster=w142, "Arm CMD.Manual Mode"=FALSE, "Arm CMD.Manual Velocity"=w141) -> (w144:T25)
        }
        frame "Manual Off Lift" {
          n234 = Unbundle By Name(w146) -> ("Rotation CMD.Lift Value"=w145:dbl)
          n235 = Bundle By Name(cluster=w146, "Lift CMD.Manual Mode"=FALSE ("Arm CMD.Manual Mode"), "Lift CMD.Manual Velocity"=w145) -> (w148:T25)
        }
        frame "Manual Off Claw Rotation" {
          n236 = Unbundle By Name(w150) -> ("Rotation CMD.Claw Rotation Value"=w149:dbl)
          n237 = Bundle By Name(cluster=w150, "Claw Rotation CMD.Manual Mode"=FALSE ("Arm CMD.Manual Mode"), "Claw Rotation CMD.Manual Velocity"=w149) -> (w152:T25)
        }
        frame "Manual Off All" {
          n238 = Unbundle By Name(w156) -> ("Rotation CMD.Arm Value"=w153:dbl, "Rotation CMD.Claw Rotation Value"=w154:dbl, "Rotation CMD.Lift Value"=w155:dbl)
          n239 = Bundle By Name(cluster=w156, "Arm CMD.Manual Mode"=FALSE, "Claw Rotation CMD.Manual Mode"=FALSE, "Lift CMD.Manual Mode"=FALSE, "Arm CMD.Manual Velocity"=w153, "Claw Rotation CMD.Manual Velocity"=w154, "Lift CMD.Manual Velocity"=w155) -> (w160:T25)
        }
        frame "Reset Stage Counter" {
          n240 = Bundle By Name(cluster=w163, "Stage Counter"=0) -> (w162:T25)
        }
        frame "Increment Counter" {
          n241 = in-place {
            n242 = in-place-cluster #1(w165) -> ("Stage Counter"=w166:i32)
            n243 = Increment(x=w166) -> (x+1=w167:i32)
            n244 = in-place-cluster #1("Stage Counter"=w167) -> (w164:T25)
          }
        }
        frame "Manual Override" {
          w168 = TRUE
          n245 = Bundle By Name(cluster=w170, "Arm CMD.Manual Override"=w168, "Claw Rotation CMD.Manual Override"=w168, "Lift CMD.Manual Override"=w168) -> (w169:T25)
        }
        frame "Manual Override Off" {
          w171 = FALSE
          n246 = Bundle By Name(cluster=w173, "Arm CMD.Manual Override"=w171, "Claw Rotation CMD.Manual Override"=w171, "Lift CMD.Manual Override"=w171) -> (w172:T25)
        }
        frame "Netural Path - Arm First" {
          n247 = Bundle By Name(cluster=w176, "Neutral Path"=TRUE) -> (w175:T25)
        }
        frame "Neutral Path - Normal" {
          n248 = Bundle By Name(cluster=w179, "Neutral Path"=FALSE) -> (w178:T25)
        }
      }
    }
    n249 = Unbundle By Name(w53) -> ("Rotation CMD"=→"Rotation CMD":T8, "Arm CMD"=→"Arm CMD":T6, "Claw Rotation CMD"=→"Claw Rotation CMD":T4, "Lift CMD"=→"Lift CMD":T2, "Stage Counter"=→"Stage Counter":i32, "State"=→"State":T1)
    n250 = Unbundle By Name(w53) -> ("Arm CMD"=w46:T6, "Claw Rotation CMD"=w45:T4, "Lift CMD"=w44:T2)
    n251 = Unbundle By Name(w53) -> ("Cycle Time(S)"=→"Cycle Time (S)":dbl)
    n252 = global write "Global_CMD.vi" "CMD_SM_Claw_Rotation"(w45) -> ()
    n253 = global write "Global_CMD.vi" "CMD_SM_Arm"(w46) -> ()
    n254 = global write "Global_CMD.vi" "CMD_SM_Lift"(w44) -> ()
  }
